vi "generic_reply.vi"(5 "Status (Error)":T1, 7 "info string":string="default", 9 "(error code)":string="default", 11 "error in (no error)":errorcluster) -> (6 "multipart message":string[](array[string]), 14 "Debug info":string, 15 "error out":errorcluster)   [LabVIEW 2019, in "mmW_commands.lvlib"]
uses:
  mmW_commands.lvlib
  TypeDefs/commands.ctl
  reply_statuscode.ctl
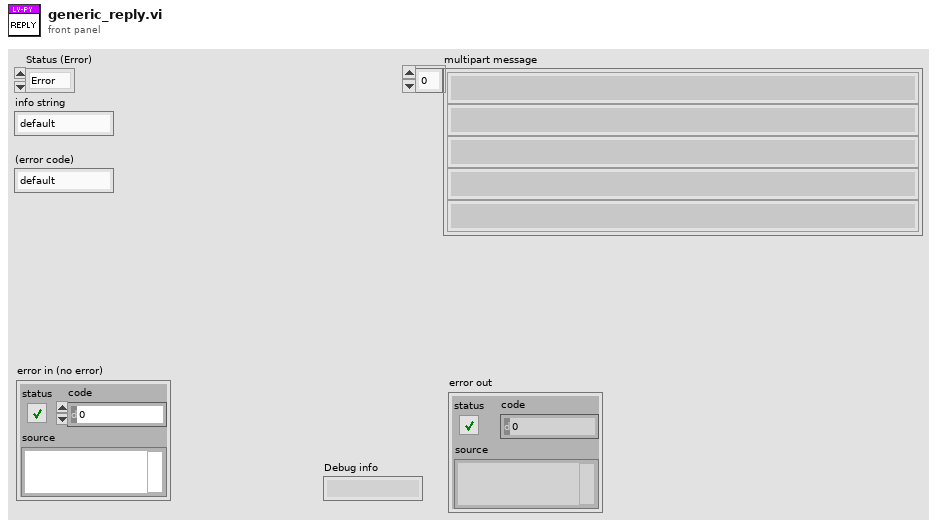
[diagram p1: front panel]
types:
  T1 = typedef "mmW_commands.lvlib/reply_statuscode.ctl" = enum16{"Error", "OK"}
  T2 = typedef "mmW_commands.lvlib/commands.ctl" = enum16{"configure_fs", "configure_rf", "configure_trigger", "equalization_enable", "equalization_start", "lo_sync_enable", "equalization_stop", "get_instrument_status", "get_versions", "initialize_hw", "pop_rx", "set_log_level", "Shutdown", "start", "start_instrument_app", "stop", "trans", "transceive", "trigger_burst", "trigger_sync_enable", "Write TX", "resp_generic", "resp_waveform", "send_trigger", "fetch", "transceive2"}
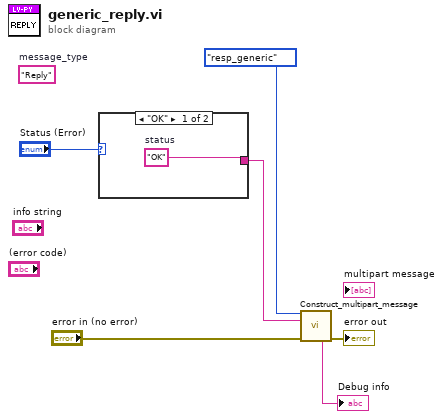
[diagram p0: block diagram]
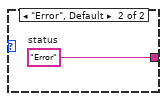
[diagram p2: hidden frame]
diagram:
  (unwired) "Reply"  # message_type
  n1 = case shown="\"OK\"" "Status (Error)" {
    tunnel: [w7 w8] -> w3
    frame "OK" {
      w7 = "OK"  # status
    }
    frame "Error", Default {
      w8 = "Error"  # status
    }
  }
  n2 = call "Construct_multipart_message.vi"("command"=commands."resp_generic", "parameters (JSON)"=w3, "error in (no error)"="error in (no error)") -> ("Debug info"=→"Debug info":string, "error out"=→"error out":errorcluster)  [unwired: 9 in, 2 out]
